vi "dfd_FXP PtByPt Direct IIR II Transposed.vi"(6 "state in":i64[](array[numeric]), 7 "quantizers":T5[](array[typedef]) {"source" items=["Coef a/k"=0, "Coef b/v"=7, "Input"=1, "Output"=2, "Multiplicand"=3, "Product"=4, "Sum"=5, "Delay"=6, "Gain"=8]}, 8 "filtering statistics in":T4(array[cluster]) {"statistics information"."min value" format="%.2f"; "statistics information"."max value" format="%.2f"; "Quantizer Source" items=["Coefficients a/k"=0, "Coefficients b/v"=7, "Input"=1, "Output"=2, "Multiplicand"=3, "Product"=4, "Sum"=5, "Delay"=6]}, 9 "coef a[1..N]":T1, 10 "coef b[0..M]":T1, 11 "x":T7={"value"=0, "wl"=0, "iwl"=0, "Signed"=TRUE} {"value" format="%.0x"}) -> (0 "filtering statistics out":T4(array[cluster]) {"statistics information"."min value" format="%.2f"; "statistics information"."max value" format="%.2f"; "Quantizer Source" items=["Coefficients a/k"=0, "Coefficients b/v"=7, "Input"=1, "Output"=2, "Multiplicand"=3, "Product"=4, "Sum"=5, "Delay"=6]}, 3 "filtered x":T7={"value"=0, "wl"=0, "iwl"=0, "Signed"=TRUE} {"value" format="%.0x"}, 4 "state out":i64[](array[numeric]))   [LabVIEW 2017, in "NI_DigFilter_FXP.lvlib"]
uses:
  <vilib>/addons/Digital Filter Design/NI_DigFilter_FXP.lvlib
  <vilib>/addons/Digital Filter Design/_Objects.llb/dfd_DFXP Data Type (scaler).ctl
  <vilib>/addons/Digital Filter Design/_Objects.llb/dfd_DFXP Operation Parameter.ctl
  <vilib>/addons/Digital Filter Design/_Objects.llb/dfd_Internal Quantization Srcs.ctl
  <vilib>/addons/Digital Filter Design/_Objects.llb/dfd_DFXP Data Type (vector).ctl
  <vilib>/addons/Digital Filter Design/_Objects.llb/DFD Quantization Sources.ctl
  <vilib>/addons/Digital Filter Design/_Objects.llb/DFD FXP Statistics Data.ctl
  <vilib>/addons/Digital Filter Design/NI_DigFilterLicensed.lvlib
panel:
  in  "DFXP array data type":T1
  in  "states":T1
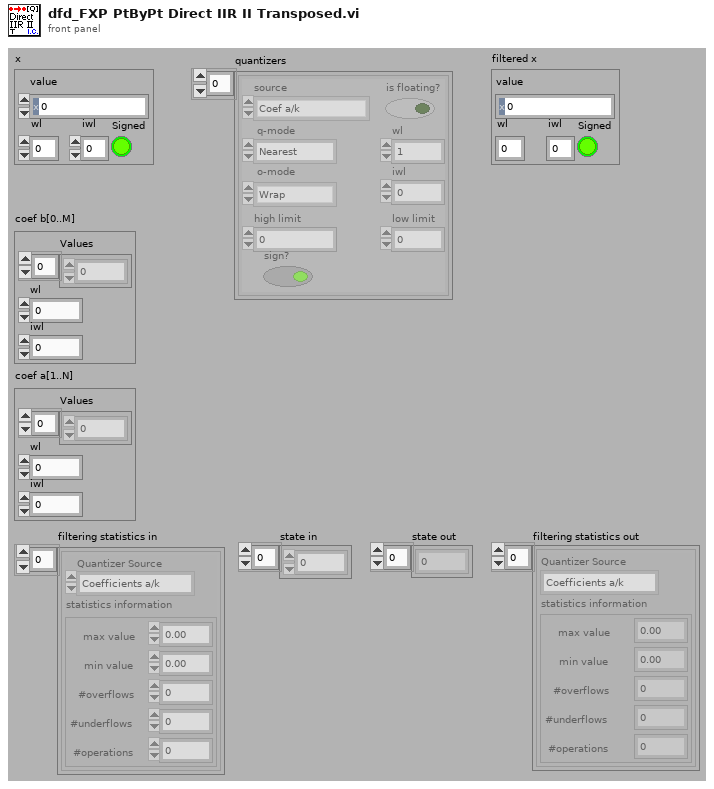
[diagram p1: front panel]
types:
  T1 = typedef "dfd_DFXP Data Type (vector).ctl" = cluster{"Values":i64[], "wl":i16, "iwl":i16}
  T2 = typedef "NI_DigFilterLicensed.lvlib/DFD Quantization Sources.ctl" = u16
  T3 = typedef "NI_DigFilterLicensed.lvlib/DFD FXP Statistics Data.ctl" = cluster{"max value":ext, "min value":ext, "#overflows":i32, "#underflows":i32, "#operations":i32}
  T4 = cluster{"Quantizer Source":T2, "statistics information":T3}[]
  T5 = typedef "dfd_DFXP Operation Parameter.ctl" = cluster{"source":T6, "is floating?":bool, "o-mode":enum16{"Saturation", "Wrap"}, "q-mode":enum16{"Nearest", "Truncation"}, "wl":i16, "high limit":i64, "low limit":i64, "iwl":i16, "sign?":bool}
  T6 = typedef "NI_DigFilterLicensed.lvlib/dfd_Internal Quantization Srcs.ctl" = u16
  T7 = typedef "dfd_DFXP Data Type (scaler).ctl" = cluster{"value":i64, "wl":i16, "iwl":i16, "Signed":bool}
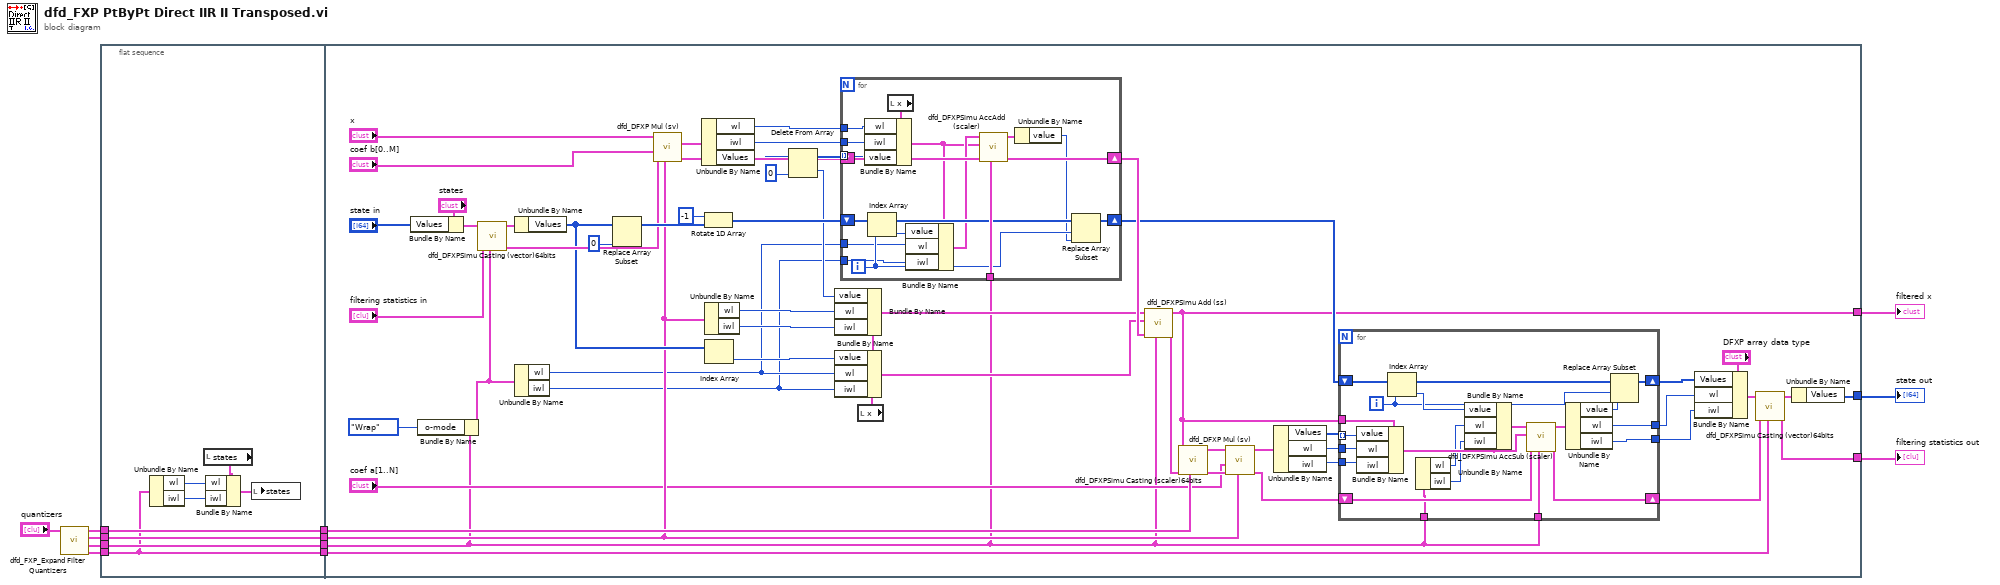
[diagram p0: block diagram]
diagram:
  n1 = call <vilib>:"dfd_FXP_Expand Filter Quantizers.vi"("FXPOPs"="quantizers") -> ("Delay"=w10:T5, "Sum"=w6:T5, "Product"=w7:T5, "Multiplicand"=w11:T5)  [unwired: 7 out]
  n2 = flat-sequence {
    tunnel: w6 -> [w18]
    tunnel: w7 -> [w19]
    tunnel: w10 -> [w13]
    tunnel: w11 -> [w20]
    tunnel: [w20] -> w4
    tunnel: [w13] -> w3
    tunnel: [w19] -> w2
    tunnel: [w18] -> w1
    tunnel: [w72] -> w9
    tunnel: [w32] -> w8
    tunnel: [w23] -> w5
    tunnel: w4 -> [w76]
    tunnel: w3 -> [w75]
    tunnel: w2 -> [w44]
    tunnel: w1 -> [w21]
    frame #0 {
      n3 = Unbundle By Name(w13) -> ("wl"=w15:i16, "iwl"=w14:i16)
      n4 = local read "states"() -> (w17:T1)
      n5 = Bundle By Name(cluster=w17, "wl"=w15, "iwl"=w14) -> (w16:T1)
      n6 = local write "states"(w16) -> ()
    }
    frame #1 {
      n7 = Bundle By Name(cluster="states", "Values"="state in") -> (w50:T1)
      n8 = Bundle By Name(cluster=w21, "o-mode"=enum16{"Saturation", "Wrap"}."Wrap" ("o_mode")) -> (w38:T5)
      n9 = call <vilib>:"dfd_DFXPSimu Casting (vector)64bits.vi"("op params"=w38, "filtering statistics in"="filtering statistics in", "Value in"=w50) -> ("filtering statistics out"=w59:T4, "Value out"=w55:T1)  [unwired: 1 in, 6 out]
      n10 = Unbundle By Name(w55) -> ("Values"=w48:i64[])
      n11 = Unbundle By Name(w38) -> ("wl"=w37:i16, "iwl"=w36:i16)
      n12 = Replace Array Subset(array=w48, new element=i64 0 ("Bits pattern")) -> (w69:i64[])  [unwired: 1 in]
      n13 = call <vilib>:"dfd_DFXP Mul (sv).vi"("op params"=w44, "filtering statistics in"=w59, "Value in 2"="coef b[0..M]", "Value in"="x") -> ("filtering statistics out"=w61:T4, "Value out"=w46:T1)  [unwired: 1 in, 5 out]
      n14 = Unbundle By Name(w46) -> ("wl"=w40:i16, "iwl"=w39:i16, "Values"=w47:i64[])
      n15 = Rotate 1D Array(1:w69, 2:-1 ("n")) -> (0:w68:i64[])
      n16 = Unbundle By Name(w44) -> ("wl"=w43:i16, "iwl"=w42:i16)
      n17 = Index Array(array=w48) -> (element=w58:i64)  [unwired: 1 in]
      n18 = Delete From Array(array=w47, index=0) -> (deleted portion=w57:i64, array with subset deleted=w62:i64[])  [unwired: 1 in]
      n19 = for {
        tunnel: w21 -> [w113]
        tunnel: w62 -> [w106] mode=indexing
        shift-right: [w111] -> w70
        shift-left: w61 -> [w112]
        shift-right: [w109] -> w65
        shift-left: w68 -> [w110]
        tunnel: w40 -> [w103]
        tunnel: w39 -> [w102]
        tunnel: w37 -> [w99]
        tunnel: w36 -> [w98]
        i -> [w108]
        n20 = Index Array(array=w110, index=w108) -> (element=w105:i64)
        n21 = local read "x"() -> (w104:T7)
        n22 = Bundle By Name(cluster=w104, "wl"=w103, "iwl"=w102, "value"=w106) -> (w100:T7)
        n23 = Bundle By Name(cluster=w100, "value"=w105, "wl"=w99, "iwl"=w98) -> (w101:T7)
        n24 = call <vilib>:"dfd_DFXPSimu AccAdd (scaler).vi"("op params"=w113, "filtering statistics in"=w112, "addend"=w100, "acc in"=w101) -> ("filtering statistics out"=w111:T4, "acc out"=w107:T7)  [unwired: 1 in, 5 out]
        n25 = Unbundle By Name(w107) -> ("value"=w97:i64)
        n26 = Replace Array Subset(array=w110, new element=w97, index=w108) -> (w109:i64[])
      }
      n27 = local read "x"() -> (w22:T7)
      n28 = Bundle By Name(cluster=w22, "value"=w57, "wl"=w43, "iwl"=w42) -> (w45:T7)
      n29 = Bundle By Name(cluster=w22, "value"=w58, "wl"=w37, "iwl"=w36) -> (w41:T7)
      n30 = call <vilib>:"dfd_DFXPSimu Add (ss).vi"("op params"=w21, "filtering statistics in"=w70, "value in 2"=w41, "value in 1"=w45) -> ("filtering statistics out"=w64:T4, "value out"=w32:T7)  [unwired: 6 out]
      n31 = call <vilib>:"dfd_DFXPSimu Casting (scaler)64bits.vi"("op params"=w76, "filtering statistics in"=w64, "Value in"=w32) -> ("filtering statistics out"=w66:T4, "Value out"=w35:T7)  [unwired: 2 in, 5 out]
      n32 = call <vilib>:"dfd_DFXP Mul (sv).vi"("op params"=w44, "filtering statistics in"=w66, "Value in 2"="coef a[1..N]", "Value in"=w35) -> ("filtering statistics out"=w74:T4, "Value out"=w34:T1)  [unwired: 1 in, 5 out]
      n33 = Unbundle By Name(w34) -> ("Values"=w33:i64[], "wl"=w31:i16, "iwl"=w30:i16)
      n34 = for {
        tunnel: w33 -> [w96] mode=indexing
        tunnel: w21 -> [w84]
        shift-right: [w94] -> w73
        shift-left: w74 -> [w95]
        shift-right: [w91] -> w54
        shift-left: w65 -> [w92]
        tunnel: w32 -> [w88]
        tunnel: w31 -> [w87]
        tunnel: w30 -> [w86]
        tunnel: [w79] -> w25
        tunnel: [w78] -> w24
        tunnel: w21 -> [w77]
        i -> [w89]
        n35 = Bundle By Name(cluster=w88, "value"=w96, "wl"=w87, "iwl"=w86) -> (w83:T7)
        n36 = Index Array(array=w92, index=w89) -> (element=w93:i64)
        n37 = Unbundle By Name(w77) -> ("wl"=w81:i16, "iwl"=w80:i16)
        n38 = Bundle By Name(cluster=w83, "value"=w93, "wl"=w81, "iwl"=w80) -> (w85:T7)
        n39 = call <vilib>:"dfd_DFXPSimu AccSub (scaler).vi"("op params"=w84, "filtering statistics in"=w95, "addend"=w83, "acc in"=w85) -> ("filtering statistics out"=w94:T4, "acc out"=w90:T7)  [unwired: 1 in, 5 out]
        n40 = Unbundle By Name(w90) -> ("value"=w82:i64, "wl"=w79:i16, "iwl"=w78:i16)
        n41 = Replace Array Subset(array=w92, new element=w82, index=w89) -> (w91:i64[])
      }
      n42 = Bundle By Name(cluster="DFXP array data type", "Values"=w54, "wl"=w25, "iwl"=w24) -> (w26:T1)
      n43 = call <vilib>:"dfd_DFXPSimu Casting (vector)64bits.vi"("op params"=w75, "filtering statistics in"=w73, "Value in"=w26) -> ("filtering statistics out"=w72:T4, "Value out"=w53:T1)  [unwired: 1 in, 6 out]
      n44 = Unbundle By Name(w53) -> ("Values"=w23:i64[])
    }
  }
  "state out" <- w5
  "filtered x" <- w8
  "filtering statistics out" <- w9
